vi "конвертюга.vi"(11 "Numeric":i32) -> (3 "Boolean":bool)   [LabVIEW 2016, in "Library.lvlib"]
uses:
  Granule-2000AT/PC/Library.lvlib
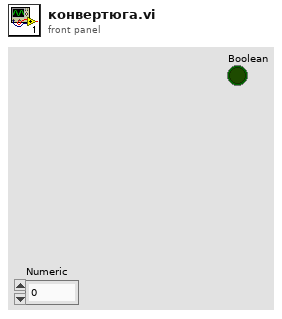
[diagram p1: front panel]
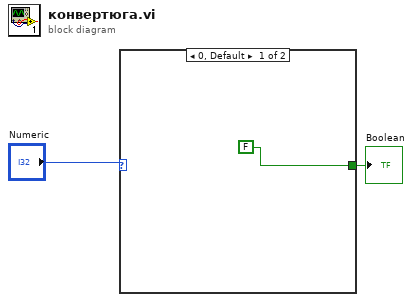
[diagram p0: block diagram]
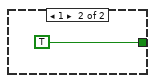
[diagram p2: hidden frame]
diagram:
  n1 = case shown="0, Default" "Numeric" {
    tunnel: [FALSE TRUE] -> w1
    frame 0, Default {
    }
    frame 1 {
    }
  }
  "Boolean" <- w1
